vi "Sensor Group 6 to Sensor Group 6 (graphical).vi"(3 "Net Angle (deg)":i32, 4 "Net Dist (mm)":i32, 6 "iRobot Sensor Group 6":T1={"Bumps + Wheel Drops"={"Wheeldrop Caster"=FALSE, "Wheeldrop Left"=FALSE, "Wheeldrop Right"=FALSE, "Bump Left"=FALSE, "Bump Right"=FALSE}, "Wall"=FALSE, "Cliff Left"=FALSE, "Cliff Front Left"=FALSE, "Cliff Front Right"=FALSE, "Cliff Right"=FALSE, "Virtual Wall"=FALSE, "Low-Side Driver + Wheel Overcurrent"={"Low-Side Driver 0"=FALSE, "Low-Side Driver 1"=FALSE, "Low-Side Driver 2"=FALSE, "Left Wheel"=FALSE, "Right Wheel"=FALSE}, "Infrared"=255, "Buttons"={"Advance"=FALSE, "Play"=FALSE}, "Distance (mm)"=0, "Angle (deg)"=0, "Charging State"=enum."Not Charging", "Voltage (mV)"=0, "Current (mA)"=0, "Battery Temperature (deg C)"=0, "Battery Charge (mAh)"=0, "Battery Capacity (mAh)"=0, "Wall Signal (0-4095)"=0, "Cliff Left Signal (0-4095)"=0, "Cliff Front Left Signal (0-4095)"=0, "Cliff Front Right Signal (0-4095)"=0, "Cliff Right Signal (0-4095)"=0, "Cargo Bay Digital Inputs"={"Digital Input 0"=FALSE, "Digital Input 1"=FALSE, "Digital Input 2"=FALSE, "Digital Input 3"=FALSE, "Device Detect"=FALSE}, "Cargo Bay Analog Signal (0-1023)"=0, "Charging Sources Available"={"Internal Charger"=FALSE, "Home Base"=FALSE}, "OI Mode"=enum."Off", "Song Number"=0, "Song Playing"=FALSE, "Number of Stream Packets"=0, "Requested Velocity (mm/s)"=0, "Requested Radius (mm)"=0, "Requested Right Wheel Velocity (mm/s)"=0, "Requested Left Wheel Velocity (mm/s)"=0} {"Infrared" format="%02x"}) -> (1 "iRobot Sensors (graphical)":T9={"Caster Wheel Drop"=FALSE, "Left Wheel Drop"=FALSE, "Right Wheel Drop"=FALSE, "Left Bump"=FALSE, "Right Bump"=FALSE, "Left Cliff"=FALSE, "Front Left Cliff"=FALSE, "Front Right Cliff"=FALSE, "Right Cliff"=FALSE, "Wall"=FALSE, "Left Wheel Overcurrent"=FALSE, "Right Wheel Overcurrent"=FALSE, "Infrared"=255, "Play"=FALSE, "Advance"=FALSE, "Net Dist (mm)"=0, "Net Angle (deg)"=0, "Charging State"=enum."Not Charging", "Voltage (mV)"=0, "Current (mA)"=0, "Battery Temperature (C)"=0, "Battery Charge (mAh)"=0, "Battery Capacity (mAh)"=255, "Wall (mm)"=0, "Left Cliff"=0, "Front Left Cliff"=0, "Front Right Cliff"=0, "Right Cliff"=0, "OI Mode"=enum."Off", "Song Number"=0, "Song Playing"=FALSE, "Power"=FALSE, "Left Wheel (mm/s)"=0, "Right Wheel (mm/s)"=0} {"Infrared" format="%02x"; "Right Wheel (mm/s)" scale=-500.0..500.0; "Left Wheel (mm/s)" scale=-500.0..500.0})   [LabVIEW 2013]
uses:
  Sensor Group 6 (graphical).ctl
  Charging State.ctl
  OI Mode.ctl
  Sensor Group 6.ctl
  Bumps + Wheel Drops.ctl
  Low-Side Driver + Wheel Overcurrent.ctl
  Buttons.ctl
  Cargo Bay Digital Inputs.ctl
  Charging Sources Available.ctl
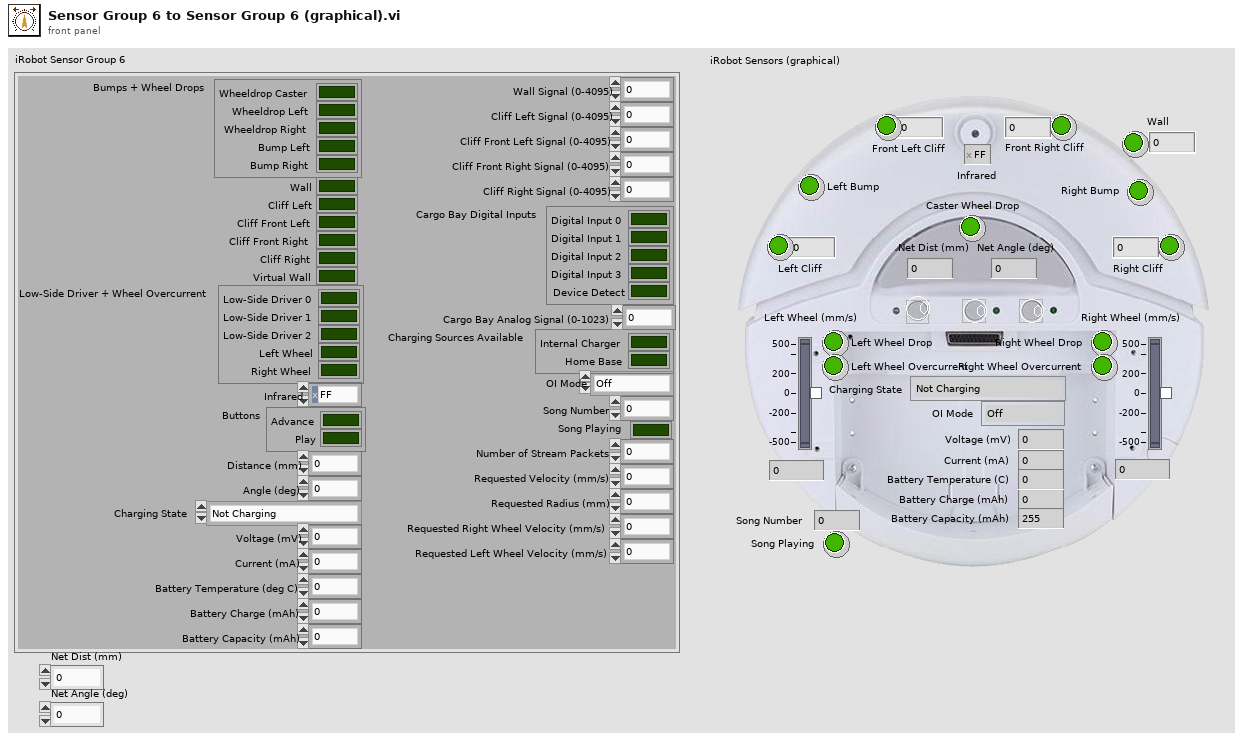
[diagram p1: front panel]
types:
  T1 = typedef "Sensor Group 6.ctl" = cluster{"Bumps + Wheel Drops":T2, "Wall":bool, "Cliff Left":bool, "Cliff Front Left":bool, "Cliff Front Right":bool, "Cliff Right":bool, "Virtual Wall":bool, "Low-Side Driver + Wheel Overcurrent":T3, "Infrared":u8, "Buttons":T4, "Distance (mm)":i32, "Angle (deg)":i32, "Charging State":T5, "Voltage (mV)":u16, "Current (mA)":i16, "Battery Temperature (deg C)":i8, "Battery Charge (mAh)":u16, "Battery Capacity (mAh)":u16, "Wall Signal (0-4095)":u16, "Cliff Left Signal (0-4095)":u16, "Cliff Front Left Signal (0-4095)":u16, "Cliff Front Right Signal (0-4095)":u16, "Cliff Right Signal (0-4095)":u16, "Cargo Bay Digital Inputs":T6, "Cargo Bay Analog Signal (0-1023)":u16, "Charging Sources Available":T7, "OI Mode":T8, "Song Number":u8, "Song Playing":bool, "Number of Stream Packets":u8, "Requested Velocity (mm/s)":i16, "Requested Radius (mm)":i16, "Requested Right Wheel Velocity (mm/s)":i16, "Requested Left Wheel Velocity (mm/s)":i16}
  T2 = typedef "Bumps + Wheel Drops.ctl" = cluster{"Wheeldrop Caster":bool, "Wheeldrop Left":bool, "Wheeldrop Right":bool, "Bump Left":bool, "Bump Right":bool}
  T3 = typedef "Low-Side Driver + Wheel Overcurrent.ctl" = cluster{"Low-Side Driver 0":bool, "Low-Side Driver 1":bool, "Low-Side Driver 2":bool, "Left Wheel":bool, "Right Wheel":bool}
  T4 = typedef "Buttons.ctl" = cluster{"Advance":bool, "Play":bool}
  T5 = typedef "Charging State.ctl" = enum16{"Not Charging", "Reconditioning Charging", "Full Charging", "Trickle Charging", "Waiting", "Charging Fault Condition"}
  T6 = typedef "Cargo Bay Digital Inputs.ctl" = cluster{"Digital Input 0":bool, "Digital Input 1":bool, "Digital Input 2":bool, "Digital Input 3":bool, "Device Detect":bool}
  T7 = typedef "Charging Sources Available.ctl" = cluster{"Internal Charger":bool, "Home Base":bool}
  T8 = typedef "OI Mode.ctl" = enum16{"Off", "Passive", "Safe", "Full"}
  T9 = typedef "Sensor Group 6 (graphical).ctl" = cluster{"Caster Wheel Drop":bool, "Left Wheel Drop":bool, "Right Wheel Drop":bool, "Left Bump":bool, "Right Bump":bool, "Left Cliff":bool, "Front Left Cliff":bool, "Front Right Cliff":bool, "Right Cliff":bool, "Wall":bool, "Left Wheel Overcurrent":bool, "Right Wheel Overcurrent":bool, "Infrared":u8, "Play":bool, "Advance":bool, "Net Dist (mm)":i32, "Net Angle (deg)":i32, "Charging State":T5, "Voltage (mV)":u16, "Current (mA)":i16, "Battery Temperature (C)":i8, "Battery Charge (mAh)":u16, "Battery Capacity (mAh)":u16, "Wall (mm)":u16, "Left Cliff":u16, "Front Left Cliff":u16, "Front Right Cliff":u16, "Right Cliff":u16, "OI Mode":T8, "Song Number":u8, "Song Playing":bool, "Power":bool, "Left Wheel (mm/s)":i16, "Right Wheel (mm/s)":i16}
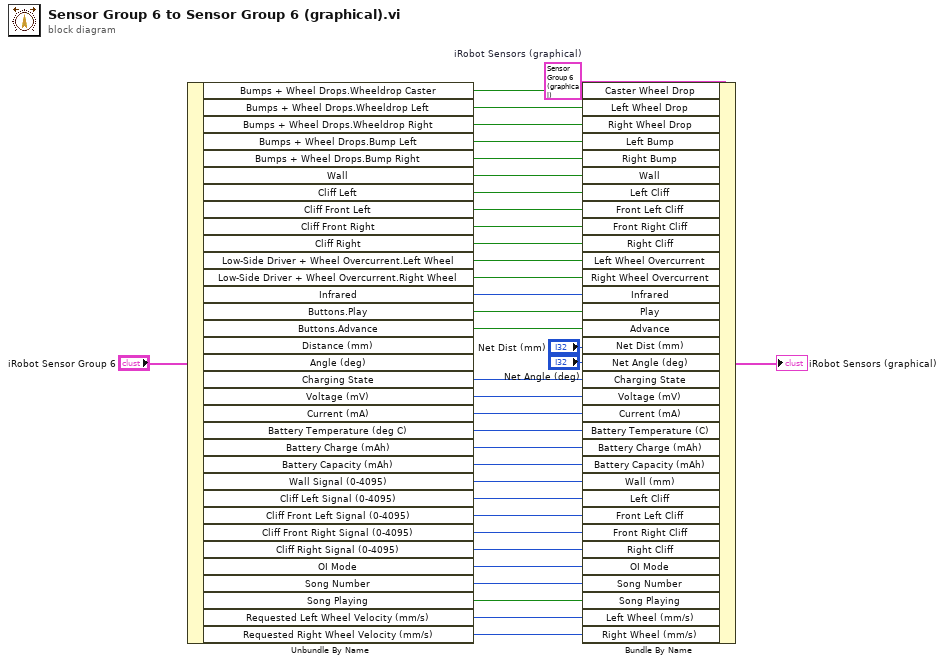
[diagram p0: block diagram]
diagram:
  w35 = T9 {"Caster Wheel Drop"=FALSE, "Left Wheel Drop"=FALSE, "Right Wheel Drop"=FALSE, "Left Bump"=FALSE, "Right Bump"=FALSE, "Left Cliff"=FALSE, "Front Left Cliff"=FALSE, "Front Right Cliff"=FALSE, "Right Cliff"=FALSE, "Wall"=FALSE, "Left Wheel Overcurrent"=FALSE, "Right Wheel Overcurrent"=FALSE, "Infrared"=0, "Play"=FALSE, "Advance"=FALSE, "Net Dist (mm)"=0, "Net Angle (deg)"=0, "Charging State"=enum."Not Charging", "Voltage (mV)"=0, "Current (mA)"=0, "Battery Temperature (C)"=0, "Battery Charge (mAh)"=0, "Battery Capacity (mAh)"=0, "Wall (mm)"=0, "Left Cliff"=0, "Front Left Cliff"=0, "Front Right Cliff"=0, "Right Cliff"=0, "OI Mode"=enum."Off", "Song Number"=0, "Song Playing"=FALSE, "Power"=FALSE, "Left Wheel (mm/s)"=0, "Right Wheel (mm/s)"=0}  # iRobot Sensors (graphical)
  n1 = Unbundle By Name("iRobot Sensor Group 6") -> ("Bumps + Wheel Drops.Wheeldrop Caster"=w34:bool, "Bumps + Wheel Drops.Wheeldrop Left"=w33:bool, "Bumps + Wheel Drops.Wheeldrop Right"=w32:bool, "Bumps + Wheel Drops.Bump Left"=w31:bool, "Bumps + Wheel Drops.Bump Right"=w30:bool, "Wall"=w29:bool, "Cliff Left"=w28:bool, "Cliff Front Left"=w27:bool, "Cliff Front Right"=w26:bool, "Cliff Right"=w25:bool, "Low-Side Driver + Wheel Overcurrent.Left Wheel"=w24:bool, "Low-Side Driver + Wheel Overcurrent.Right Wheel"=w23:bool, "Infrared"=w22:u8, "Buttons.Play"=w21:bool, "Buttons.Advance"=w20:bool, "Charging State"=w19:T5, "Voltage (mV)"=w18:u16, "Current (mA)"=w17:i16, "Battery Temperature (deg C)"=w16:i8, "Battery Charge (mAh)"=w15:u16, "Battery Capacity (mAh)"=w14:u16, "Wall Signal (0-4095)"=w13:u16, "Cliff Left Signal (0-4095)"=w12:u16, "Cliff Front Left Signal (0-4095)"=w11:u16, "Cliff Front Right Signal (0-4095)"=w10:u16, "Cliff Right Signal (0-4095)"=w9:u16, "OI Mode"=w8:T8, "Song Number"=w7:u8, "Song Playing"=w6:bool, "Requested Left Wheel Velocity (mm/s)"=w5:i16, "Requested Right Wheel Velocity (mm/s)"=w4:i16)  [unwired: 2 out]
  n2 = Bundle By Name(cluster=w35, "Caster Wheel Drop"=w34, "Left Wheel Drop"=w33, "Right Wheel Drop"=w32, "Left Bump"=w31, "Right Bump"=w30, "Wall"=w29, "Left Cliff"=w28, "Front Left Cliff"=w27, "Front Right Cliff"=w26, "Right Cliff"=w25, "Left Wheel Overcurrent"=w24, "Right Wheel Overcurrent"=w23, "Infrared"=w22, "Play"=w21, "Advance"=w20, "Net Dist (mm)"="Net Dist (mm)", "Net Angle (deg)"="Net Angle (deg)", "Charging State"=w19, "Voltage (mV)"=w18, "Current (mA)"=w17, "Battery Temperature (C)"=w16, "Battery Charge (mAh)"=w15, "Battery Capacity (mAh)"=w14, "Wall (mm)"=w13, "Left Cliff"=w12, "Front Left Cliff"=w11, "Front Right Cliff"=w10, "Right Cliff"=w9, "OI Mode"=w8, "Song Number"=w7, "Song Playing"=w6, "Left Wheel (mm/s)"=w5, "Right Wheel (mm/s)"=w4) -> (→"iRobot Sensors (graphical)":T9)
